vi "Open Acrobat Manual_7_adq.vi"(4 "error in (no error)":errorcluster, 7 "acrobat document":path) -> (0 "error out":errorcluster)   [LabVIEW 2019]
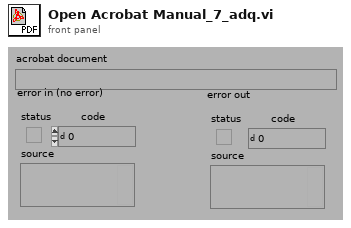
[diagram p1: front panel]
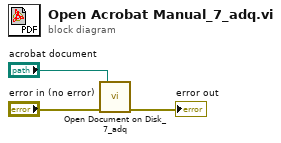
[diagram p0: block diagram]
diagram:
  n1 = call "Open Document on Disk_7_adq.vi"("error in (no error)"="error in (no error)", "document path"="acrobat document") -> ("error out"=→"error out":errorcluster)  [unwired: 5 in]
